vi "singlePressButton.vi"(11 "Boolean":bool) -> (3 "Boolean 2":bool)   [LabVIEW 2020]
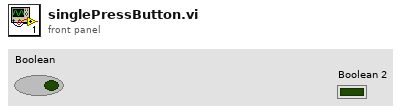
[diagram p1: front panel]
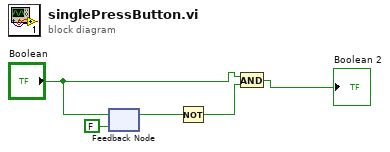
[diagram p0: block diagram]
diagram:
  n1 = feedback-in #1("Boolean") -> ()
  n2 = feedback #1(FALSE ("Boolean")) -> (w1:bool)
  n3 = Not(x=w1) -> (.not. x?=w4:bool)
  n4 = And(x="Boolean", y=w4) -> (x .and. y?=→"Boolean 2":bool)
